vi "EPS-Query Operation Status.vi"(8 "error in":errorcluster, 11 "EPS Setting In":T2) -> (0 "error out":errorcluster, 1 "OFF?":bool, 2 "Value Type":T1, 3 "EPS Setting Out":T2)   [LabVIEW 2018]
uses:
  Data Def/EPS-Setting.ctl
  Data Def/EPS-Value Type.ctl
  Data Def/EPS-Access Mode.ctl
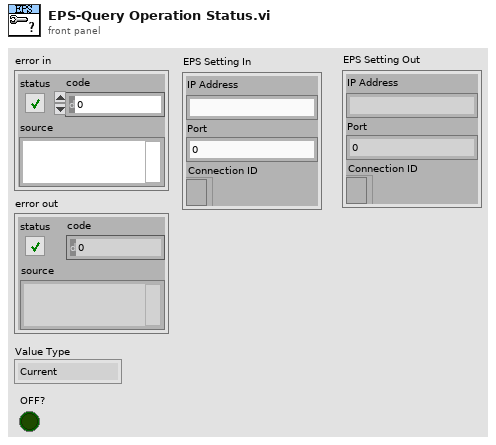
[diagram p1: front panel]
types:
  T1 = typedef "EPS-Value Type.ctl" = enum16{"Current", "Vlotage", "Power"}
  T2 = typedef "EPS-Setting.ctl" = cluster{"IP Address":string, "Port":u16, "Connection ID":refnum<k5>}
  T3 = typedef "EPS-Access Mode.ctl" = enum16{"Read", "Write"}
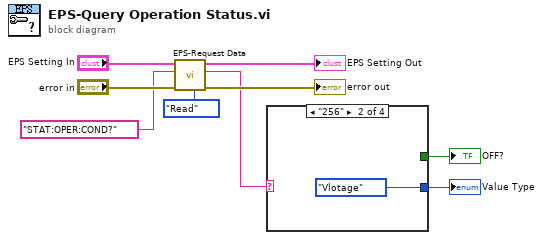
[diagram p0: block diagram]
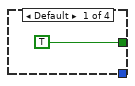
[diagram p2: hidden frame]
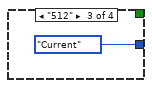
[diagram p3: hidden frame]
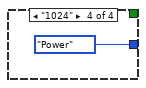
[diagram p4: hidden frame]
diagram:
  n1 = call "EPS-Request Data.vi"("Access Mode"=EPS-Access_Mode."Read", "error in"="error in", "Requst Data"="STAT:OPER:COND?", "EPS Setting In"="EPS Setting In") -> ("error out"=→"error out":errorcluster, "Response Data"=w3:string, "EPS Setting Out"=→"EPS Setting Out":T2)  [unwired: 5 in]
  n2 = case shown="\"256\"" w3 {
    tunnel: [_ EPS-Value_Type."Vlotage" ("Value Type") EPS-Value_Type."Current" ("Value Type") EPS-Value_Type."Power" ("Value Type")] -> w1
    tunnel: [TRUE _ _ _] -> w2
    frame Default {
    }
    frame "256" {
    }
    frame "512" {
    }
    frame "1024" {
    }
  }
  "Value Type" <- w1
  "OFF?" <- w2
